vi "Flatten.vi"(6 "FIFO Timestamps":T1, 8 "error in (no error)":errorcluster, 10 "Data In":refnum<data-value>[](array[refnum]), 11 "CIFTag in":refnum<class "CIF_NIChn_Fifo_Power_DVR.lvclass">) -> (0 "error out":errorcluster, 2 "Data Out":refnum<data-value>[](array[refnum]), 3 "CIFTag out":refnum<class "CIF_NIChn_Fifo_Power_DVR.lvclass">)   [LabVIEW 2021, in "CIF_NIChn_Fifo_Power_DVR.lvclass"]
uses:
  CIF_NIChn_Fifo_Power_DVR.lvclass
  ChannelCommon/typedef/TimeStamps.ctl
  ChannelCommon/typedef/Datatype Waveform.ctl
  CIF_NIChn_Fifo_Power_DVR.lvclass/CIF_NIChn_Fifo_Power_DVR.ctl
  ChannelCommon/CIFFIFO/CIFfifo.lvclass/CIFfifo.ctl
  ChannelCommon/CIFFIFO/Accessors/Write T0.vi
  ChannelCommon/CIFFIFO/Accessors/Write T_Out.vi
  ChannelCommon/CIFFIFO/Accessors/Write ClockID.vi
  <vilib>/CIF Foundation/CIF Utilities/Time/System Time/Get System Time.vi
  ChannelCommon/Utilities/Flatten Header.vi
  ChannelCommon/CIFFIFO/Flatten/DVR Flatten.vi/6fdbece9-bad6-4a8e-9bf7-fe1528478dd6.vi
  ChannelCommon/CIFFIFO/Accessors/Write Payload Length.vi
  ChannelCommon/CIFFIFO/Accessors/Read Header.vi
  <vilib>/CIF Foundation/CIF Utilities/Time/System Time/LabVIEW Time to TAI Time.vi
  CIFCore/Common/Utilities/Add Error.vi
  ChannelCommon/CIFFIFO/Flatten/DVR Flatten.vi/6fdbece9-bad6-4a8e-9bf7-fe1528478dd6.vi/c28b0ead-42ad-4072-80a2-aca7f2bd7ce3.vi
  <vilib>/CIF Foundation/CIF Utilities/Errors/Append Error Location.vi
  ChannelCommon/CIFFIFO/CIFfifo.lvclass
  ChannelCommon/ChannelCommon.lvlib
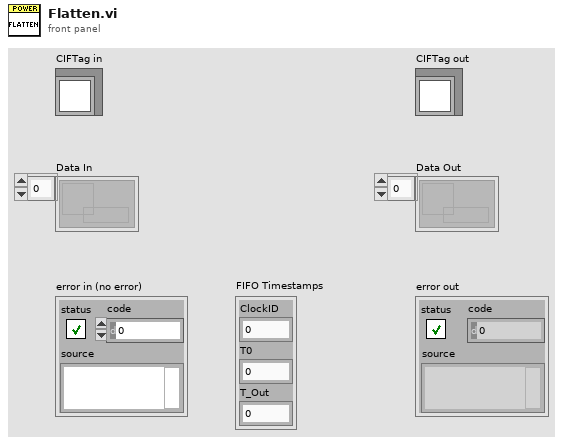
[diagram p1: front panel]
types:
  T1 = typedef "ChannelCommon.lvlib/TimeStamps.ctl" = cluster{"ClockID":u8, "T0":i64, "T_Out":i64}
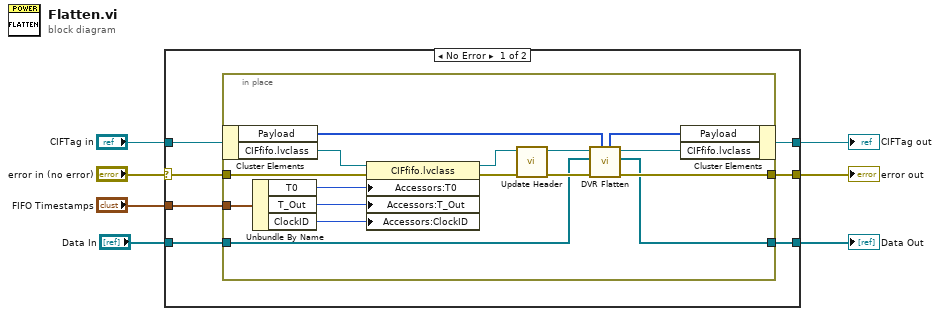
[diagram p0: block diagram]
diagram:
  n1 = case shown="No Error" "error in (no error)" {
    selector: "error in (no error)" -> [w11 w33]
    tunnel: [w14 w33] -> w6
    tunnel: [w13 w32] -> w4
    tunnel: "CIFTag in" -> [w12 w32]
    tunnel: "FIFO Timestamps" -> [w10 _]
    tunnel: "Data In" -> [w9 w31]
    tunnel: [w8 w31] -> w1
    frame No Error {
      n2 = in-place {
        in-place-border: w11 -> [w27]
        in-place-border: [w21] -> w14
        in-place-border: w10 -> [w20]
        in-place-border: w9 -> [w16]
        in-place-border: [w15] -> w8
        n3 = in-place-cluster #1(w12) -> ("Payload"=w24:u8[], "CIFfifo.lvclass"=w30:refnum<class "CIFfifo.lvclass">)
        n4 = Unbundle By Name(w20) -> ("T0"=w19:i64, "T_Out"=w18:i64, "ClockID"=w17:u8)
        n5 = property class="CIFfifo.lvclass"(reference=w30, error in=w27, "Accessors:T0"=w19, "Accessors:T_Out"=w18, "Accessors:ClockID"=w17) -> (reference out=w29:refnum<class "CIFfifo.lvclass">, error out=w28:errorcluster)
        n6 = call "Update Header.vi"("error in (no error)"=w28, "CIFFIFO in"=w29) -> ("error out"=w25:errorcluster, "CIFFIFO out"=w26:refnum<class "CIFfifo.lvclass">)  [unwired: 8 in]
        n7 = call "DVR Flatten.vi"("payload in"=w24, "error in (no error)"=w25, "Data In"=w16, "CIFFifo in"=w26) -> ("error out"=w21:errorcluster, "Data Out"=w15:refnum<data-value>[], "CIFFifo out"=w22:refnum<class "CIFfifo.lvclass">, "payload out"=w23:u8[])  [unwired: 3 in, 1 out]
        n8 = in-place-cluster #1("Payload"=w23, "CIFfifo.lvclass"=w22) -> (w13:refnum<class "CIF_NIChn_Fifo_Power_DVR.lvclass">)
      }
    }
    frame Error {
    }
  }
  "error out" <- w6
  "CIFTag out" <- w4
  "Data Out" <- w1
